vi "slow retract.vi"(7 "reset motion":T1=enum."fast", 8 "error in":errorcluster, 10 "retract distance (um)":dbl=100.0, 11 "manp in":T2={"Actuator COM"="COM6", "Actuator type"=enum."Scientifica"}) -> (0 "error out":errorcluster, 3 "manip out":T2={"Actuator COM"="COM14", "Actuator type"=enum."Scientifica"})   [LabVIEW 2015]
uses:
  controls/scope_motion.ctl
  pipette cleaning/pressure box/cleaning_soft/controls/scientifica_commands.ctl
  pipette cleaning/pressure box/cleaning_soft/controls/actuator_type.ctl
  pipette cleaning/pressure box/cleaning_soft/controls/actuator_cluster.ctl
panel:
  in  "retract step size (um)":dbl=5.0
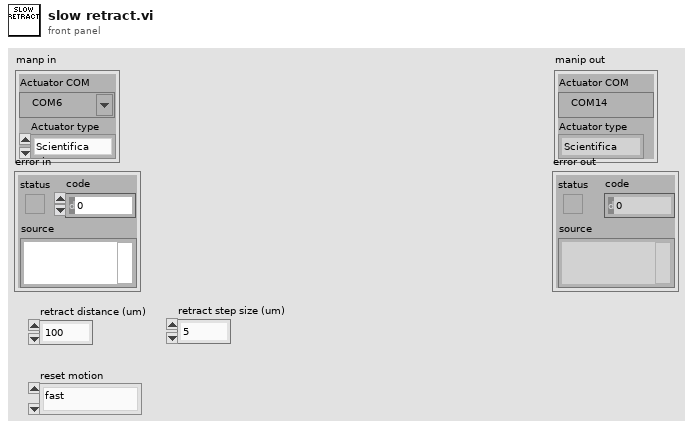
[diagram p1: front panel]
types:
  T1 = typedef "scope_motion.ctl" = enum16{"superSlow", "fast", "slow", "find slice speed", "slow_dualPatch"}
  T2 = typedef "actuator_cluster.ctl" = cluster{"Actuator COM":refnum<visa-resource-name>, "Actuator type":T3}
  T3 = typedef "actuator_type.ctl" = enum16{"Scientifica", "Sutter", "Demo", "Off"}
  T4 = typedef "scientifica_commands.ctl" = enum16{"ANGLE", "INSET", "FIRST", "ZERO", "Pz", "P", "absz", "ACC", "TOP", "STOP", "rel", "relz", "abs", "IN", "vj", "APROACH", "OBJS", "OBJU", "OUT", "OBJ", "OBJL", "SET", "OBJD", "STEP", "SETSTEP", "S", "UUX", "UUY", "UUZ"}
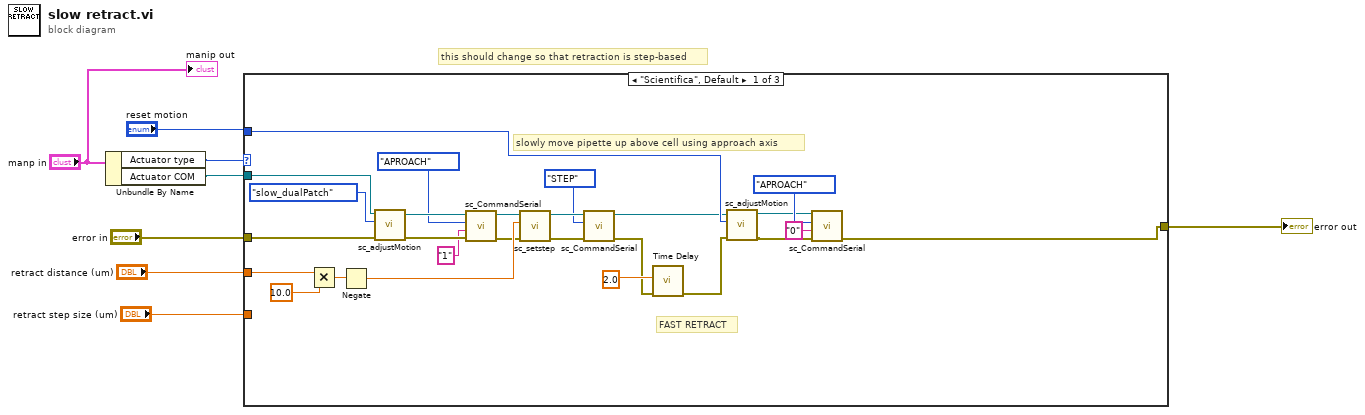
[diagram p0: block diagram]
diagram:
  # "this should change so that retraction is step-based"
  n1 = Unbundle By Name("manp in") -> ("Actuator type"=w7:T3, "Actuator COM"=w6:refnum<visa-resource-name>)
  n2 = case shown="\"Scientifica\", Default" w7 {
    tunnel: w6 -> [w31 _ _]
    tunnel: "retract distance (um)" -> [w34 _ _]
    tunnel: "error in" -> [w33 w35 w36]
    tunnel: [w32 w35 w36] -> w4
    tunnel: "reset motion" -> [w30 _ _]
    tunnel: "retract step size (um)" -> [_ _ _]
    frame "Scientifica", Default {
      # "FAST RETRACT"
      # "slowly move pipette up above cell using approach axis"
      n3 = Multiply(x=w34, y=10.0) -> (x*y=w12:dbl)
      n4 = Negate(x=w12) -> (-x=w11:dbl)
      n5 = call "sc_adjustMotion.vi"("error in (no error)"=w33, "motion"=scope_motion."slow_dualPatch", "VISA handle"=w31) -> ("error out"=w15:errorcluster, "Dup. VISA handle"=w16:refnum<visa-resource-name>)  [unwired: 7 in]
      n6 = call "sc_CommandSerial.vi"("error in (no error)"=w15, "argument"="1", "Scientifica commands"=scientifica_commands."APROACH", "VISA handle"=w16) -> ("error out"=w9:errorcluster, "Dup. VISA handle"=w10:refnum<visa-resource-name>)  [unwired: 4 in, 2 out]
      n7 = call "sc_setstep.vi"("error in"=w9, "step distance (steps)"=w11, "VISA in"=w10) -> ("error out"=w22:errorcluster, "VISA out"=w23:refnum<visa-resource-name>)  [unwired: 6 in, 1 out]
      n8 = call "sc_CommandSerial.vi"("error in (no error)"=w22, "Scientifica commands"=scientifica_commands."STEP", "VISA handle"=w23) -> ("error out"=w18:errorcluster, "Dup. VISA handle"=w21:refnum<visa-resource-name>)  [unwired: 5 in, 2 out]
      n9 = call "Time Delay"("error in (no error)"=w18, "Delay Time (s)"=2.0) -> ("error out"=w17:errorcluster)  [unwired: 9 in]
      n10 = call "sc_adjustMotion.vi"("error in (no error)"=w17, "motion"=w30, "VISA handle"=w21) -> ("error out"=w24:errorcluster, "Dup. VISA handle"=w25:refnum<visa-resource-name>)  [unwired: 7 in]
      n11 = call "sc_CommandSerial.vi"("error in (no error)"=w24, "argument"="0", "Scientifica commands"=scientifica_commands."APROACH", "VISA handle"=w25) -> ("error out"=w32:errorcluster)  [unwired: 4 in, 3 out]
    }
    frame "Sutter" {
    }
    frame "Demo" {
    }
  }
  "error out" <- w4
  "manip out" <- "manp in"
